vi "data_acquisition.vi"() -> ()   [LabVIEW 2020]
uses:
  <vilib>/regexp/Match Regular Expression.xnode
panel:
  in  "VISA resource name":refnum<visa-resource-name>="USB0::0x0471::0x2515::482A16001::INSTR"
  out "Resistance":dbl(graph)
  in  "measurement delay time (default 0.003)":dbl=0.003
  in  "Measurement speed":enum16{"FAST", "SLOW"}(ring)
  out "Samples / Second":dbl
  in  "measurement time":enum16{"FAST", "MED", "SLOW1", "SLOW2"}(ring)
  in  "Resistance measurement range":T1(ring)
  in  "Measurement mode":T2(ring)=enum."Resistance and Temp"
  in  "Display State":enum16{"Display ON", "Display OFF"}(ring)=enum."Display OFF"
  out "Temp":dbl
  out "Resistance":dbl format="%#_6p"
  out "read buffer":string
  in  "stop 2":bool
  out "error out":errorcluster
  # "Only 2 Ohm, 20 Ohm, 200 Ohm, 2 k \nare valid for  Measurement Mode at\nLow Voltage (LPR, LPR-T)"
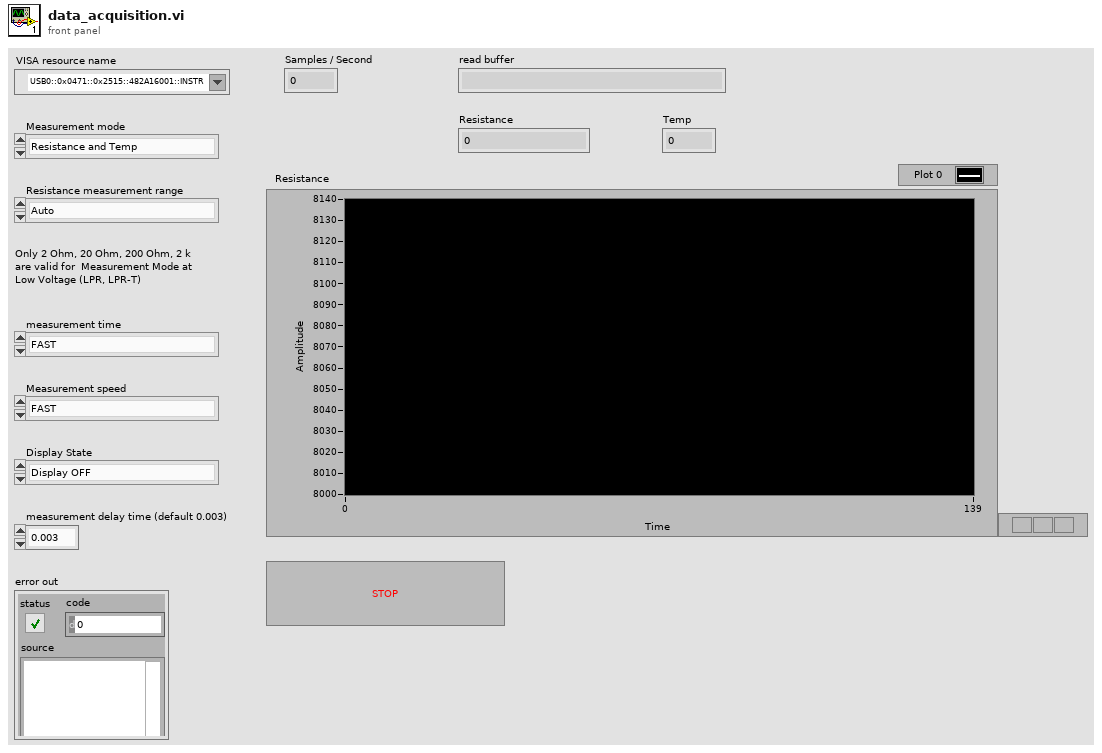
[diagram p1: front panel]
types:
  T1 = enum16{"Auto", "20 milli-Ohms", "200 milli-Ohms", "2 Ohms", "20 Ohms", "200 Ohms", "2 k-Ohms", "20 k-Ohms", "100 k-Ohms", "1 M-Ohms", "10 M-Ohms", "100 M-Ohms"}
  T2 = enum16{"Resistance", "Resistance and Temp", "Low Power Resistance", "Low Power Resisance and Temp", "Temp"}
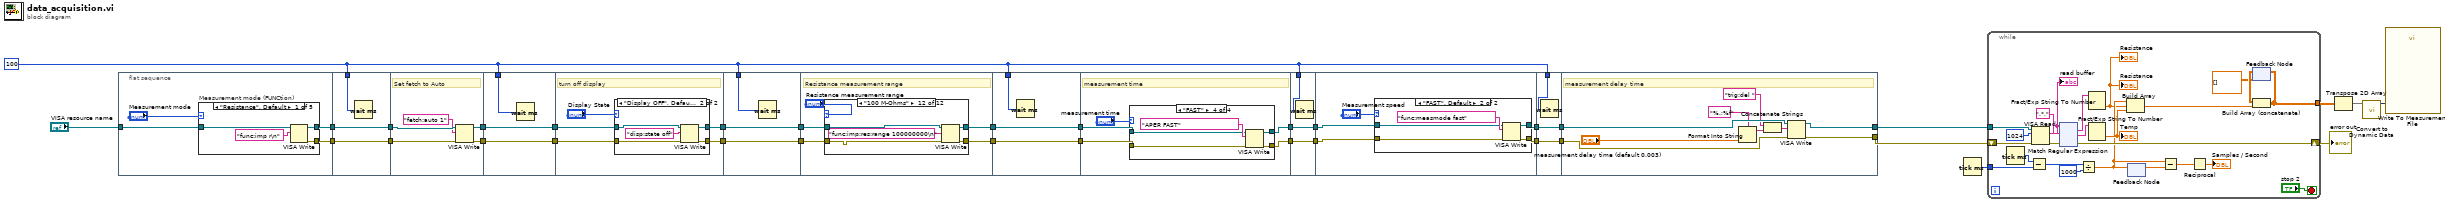
[diagram p0: block diagram]
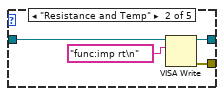
[diagram p2: hidden frame]
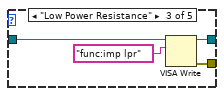
[diagram p3: hidden frame]
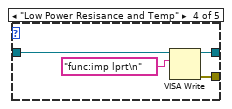
[diagram p4: hidden frame]
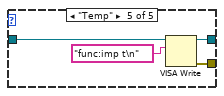
[diagram p5: hidden frame]
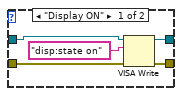
[diagram p6: hidden frame]
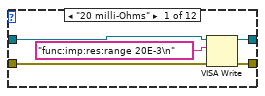
[diagram p7: hidden frame]
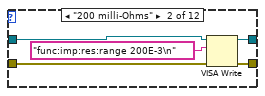
[diagram p8: hidden frame]
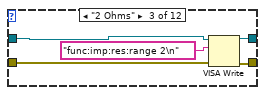
[diagram p9: hidden frame]
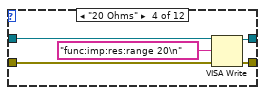
[diagram p10: hidden frame]
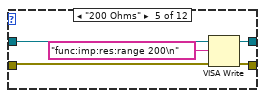
[diagram p11: hidden frame]
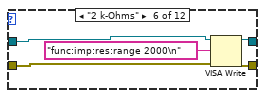
[diagram p12: hidden frame]
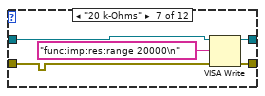
[diagram p13: hidden frame]
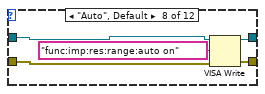
[diagram p14: hidden frame]
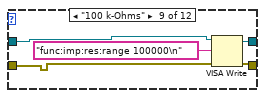
[diagram p15: hidden frame]
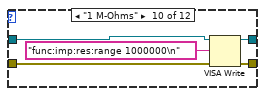
[diagram p16: hidden frame]
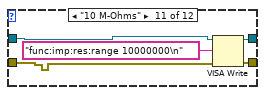
[diagram p17: hidden frame]
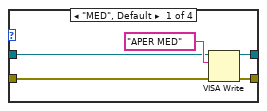
[diagram p18: hidden frame]
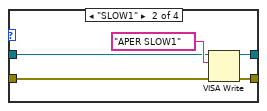
[diagram p19: hidden frame]
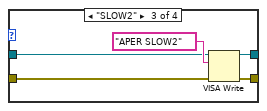
[diagram p20: hidden frame]
diagram:
  w1 = u32 100 ("delay before read (ms)")
  n1 = flat-sequence {
    tunnel: "VISA resource name" -> [w36]
    tunnel: [w34] -> w18
    tunnel: [w35] -> w17
    tunnel: [w60] -> w26
    tunnel: [w59] -> w25
    tunnel: w18 -> [w60]
    tunnel: w17 -> [w59]
    tunnel: w1 -> [w58]
    tunnel: w26 -> [w65]
    tunnel: w25 -> [w64]
    tunnel: [w63] -> w24
    tunnel: [w62] -> w23
    tunnel: w24 -> [w68]
    tunnel: w23 -> [w67]
    tunnel: w1 -> [w66]
    tunnel: [w68] -> w22
    tunnel: [w67] -> w21
    tunnel: w22 -> [w70]
    tunnel: w21 -> [w73]
    tunnel: [w72] -> w20
    tunnel: [w71] -> w19
    tunnel: w20 -> [w85]
    tunnel: w1 -> [w84]
    tunnel: w19 -> [w86]
    tunnel: [w86] -> w15
    tunnel: [w85] -> w14
    tunnel: w15 -> [w89]
    tunnel: w14 -> [w90]
    tunnel: [w87] -> w13
    tunnel: [w88] -> w12
    tunnel: w13 -> [w154]
    tunnel: w12 -> [w153]
    tunnel: [w154] -> w11
    tunnel: [w153] -> w10
    tunnel: w1 -> [w152]
    tunnel: w11 -> [w157]
    tunnel: w10 -> [w158]
    tunnel: [w155] -> w9
    tunnel: [w156] -> w8
    tunnel: w9 -> [w182]
    tunnel: w8 -> [w181]
    tunnel: [w182] -> w7
    tunnel: [w181] -> w6
    tunnel: w1 -> [w180]
    tunnel: w7 -> [w185]
    tunnel: w6 -> [w186]
    tunnel: [w184] -> w5
    tunnel: [w183] -> w4
    tunnel: w5 -> [w200]
    tunnel: w4 -> [w199]
    tunnel: [w200] -> w3
    tunnel: [w199] -> w2
    tunnel: w1 -> [w198]
    tunnel: [w206] -> w33
    tunnel: [w207] -> w32
    tunnel: w3 -> [w208]
    tunnel: w2 -> [w209]
    frame #0 {
      n2 = case "Measurement mode (FUNCtion)" shown="\"Resistance\", Default" "Measurement mode" {
        tunnel: w36 -> [w40 w45 w48 w52 w56]
        tunnel: [w39 w43 w47 w51 w55] -> w35
        tunnel: [w38 w42 w46 w50 w54] -> w34
        frame "Resistance", Default {
          n3 = VISA Write(VISA resource name=w40, write buffer="func:imp r\n") -> (VISA resource name out=w39:refnum<visa-resource-name>, error out=w38:errorcluster)  [unwired: 1 in, 1 out]
        }
        frame "Resistance and Temp" {
          n4 = VISA Write(VISA resource name=w45, write buffer="func:imp rt\n") -> (VISA resource name out=w43:refnum<visa-resource-name>, error out=w42:errorcluster)  [unwired: 1 in, 1 out]
        }
        frame "Low Power Resistance" {
          n5 = VISA Write(VISA resource name=w48, write buffer="func:imp lpr") -> (VISA resource name out=w47:refnum<visa-resource-name>, error out=w46:errorcluster)  [unwired: 1 in, 1 out]
        }
        frame "Low Power Resisance and Temp" {
          n6 = VISA Write(VISA resource name=w52, write buffer="func:imp lprt\n") -> (VISA resource name out=w51:refnum<visa-resource-name>, error out=w50:errorcluster)  [unwired: 1 in, 1 out]
        }
        frame "Temp" {
          n7 = VISA Write(VISA resource name=w56, write buffer="func:imp t\n") -> (VISA resource name out=w55:refnum<visa-resource-name>, error out=w54:errorcluster)  [unwired: 1 in, 1 out]
        }
      }
    }
    frame #1 {
      n8 = Wait (ms)(milliseconds to wait=w58) -> ()  [unwired: 1 out]
    }
    frame #2 {
      # "Set fetch to Auto"
      n9 = VISA Write(VISA resource name=w64, write buffer="fetch:auto 1", error in (no error)=w65) -> (VISA resource name out=w62:refnum<visa-resource-name>, error out=w63:errorcluster)  [unwired: 1 out]
    }
    frame #3 {
      n10 = Wait (ms)(milliseconds to wait=w66) -> ()  [unwired: 1 out]
    }
    frame #4 {
      # "turn off display"
      n11 = case shown="\"Display OFF\", Default" "Display State" {
        tunnel: w73 -> [w74 w82]
        tunnel: [w75 w81] -> w72
        tunnel: [w76 w80] -> w71
        tunnel: w70 -> [w77 w79]
        frame "Display ON" {
          n12 = VISA Write(VISA resource name=w74, write buffer="disp:state on", error in (no error)=w77) -> (VISA resource name out=w75:refnum<visa-resource-name>, error out=w76:errorcluster)  [unwired: 1 out]
        }
        frame "Display OFF", Default {
          n13 = VISA Write(VISA resource name=w82, write buffer="disp:state off", error in (no error)=w79) -> (VISA resource name out=w81:refnum<visa-resource-name>, error out=w80:errorcluster)  [unwired: 1 out]
        }
      }
    }
    frame #5 {
      n14 = Wait (ms)(milliseconds to wait=w84) -> ()  [unwired: 1 out]
    }
    frame #6 {
      # "Resistance measurement range"
      n15 = case shown="\"100 M-Ohms\"" "Resistance measurement range" {
        tunnel: w90 -> [w92 w100 w105 w108 w115 w117 w122 w127 w134 w137 w142 w148]
        tunnel: [w93 w99 w102 w110 w113 w120 w125 w130 w132 w140 w145 w150] -> w88
        tunnel: [w94 w98 w103 w109 w112 w119 w124 w129 w135 w139 w144 w149] -> w87
        tunnel: w89 -> [w95 w97 w104 w107 w114 w118 w123 w128 w133 w138 w143 w147]
        frame "20 milli-Ohms" {
          n16 = VISA Write(VISA resource name=w92, write buffer="func:imp:res:range 20E-3\n", error in (no error)=w95) -> (VISA resource name out=w93:refnum<visa-resource-name>, error out=w94:errorcluster)  [unwired: 1 out]
        }
        frame "200 milli-Ohms" {
          n17 = VISA Write(VISA resource name=w100, write buffer="func:imp:res:range 200E-3\n", error in (no error)=w97) -> (VISA resource name out=w99:refnum<visa-resource-name>, error out=w98:errorcluster)  [unwired: 1 out]
        }
        frame "2 Ohms" {
          n18 = VISA Write(VISA resource name=w105, write buffer="func:imp:res:range 2\n", error in (no error)=w104) -> (VISA resource name out=w102:refnum<visa-resource-name>, error out=w103:errorcluster)  [unwired: 1 out]
        }
        frame "20 Ohms" {
          n19 = VISA Write(VISA resource name=w108, write buffer="func:imp:res:range 20\n", error in (no error)=w107) -> (VISA resource name out=w110:refnum<visa-resource-name>, error out=w109:errorcluster)  [unwired: 1 out]
        }
        frame "200 Ohms" {
          n20 = VISA Write(VISA resource name=w115, write buffer="func:imp:res:range 200\n", error in (no error)=w114) -> (VISA resource name out=w113:refnum<visa-resource-name>, error out=w112:errorcluster)  [unwired: 1 out]
        }
        frame "2 k-Ohms" {
          n21 = VISA Write(VISA resource name=w117, write buffer="func:imp:res:range 2000\n", error in (no error)=w118) -> (VISA resource name out=w120:refnum<visa-resource-name>, error out=w119:errorcluster)  [unwired: 1 out]
        }
        frame "20 k-Ohms" {
          n22 = VISA Write(VISA resource name=w122, write buffer="func:imp:res:range 20000\n", error in (no error)=w123) -> (VISA resource name out=w125:refnum<visa-resource-name>, error out=w124:errorcluster)  [unwired: 1 out]
        }
        frame "Auto", Default {
          n23 = VISA Write(VISA resource name=w127, write buffer="func:imp:res:range:auto on", error in (no error)=w128) -> (VISA resource name out=w130:refnum<visa-resource-name>, error out=w129:errorcluster)  [unwired: 1 out]
        }
        frame "100 k-Ohms" {
          n24 = VISA Write(VISA resource name=w134, write buffer="func:imp:res:range 100000\n", error in (no error)=w133) -> (VISA resource name out=w132:refnum<visa-resource-name>, error out=w135:errorcluster)  [unwired: 1 out]
        }
        frame "1 M-Ohms" {
          n25 = VISA Write(VISA resource name=w137, write buffer="func:imp:res:range 1000000\n", error in (no error)=w138) -> (VISA resource name out=w140:refnum<visa-resource-name>, error out=w139:errorcluster)  [unwired: 1 out]
        }
        frame "10 M-Ohms" {
          n26 = VISA Write(VISA resource name=w142, write buffer="func:imp:res:range 10000000\n", error in (no error)=w143) -> (VISA resource name out=w145:refnum<visa-resource-name>, error out=w144:errorcluster)  [unwired: 1 out]
        }
        frame "100 M-Ohms" {
          n27 = VISA Write(VISA resource name=w148, write buffer="func:imp:res:range 100000000\n", error in (no error)=w147) -> (VISA resource name out=w150:refnum<visa-resource-name>, error out=w149:errorcluster)  [unwired: 1 out]
        }
      }
    }
    frame #7 {
      n28 = Wait (ms)(milliseconds to wait=w152) -> ()  [unwired: 1 out]
    }
    frame #8 {
      # "measurement time"
      n29 = case shown="\"FAST\"" "measurement time" {
        tunnel: w158 -> [w160 w168 w173 w175]
        tunnel: [w161 w167 w170 w178] -> w156
        tunnel: [w162 w166 w171 w177] -> w155
        tunnel: w157 -> [w163 w165 w172 w176]
        frame "MED", Default {
          n30 = VISA Write(VISA resource name=w160, write buffer="APER MED", error in (no error)=w163) -> (VISA resource name out=w161:refnum<visa-resource-name>, error out=w162:errorcluster)  [unwired: 1 out]
        }
        frame "SLOW1" {
          n31 = VISA Write(VISA resource name=w168, write buffer="APER SLOW1", error in (no error)=w165) -> (VISA resource name out=w167:refnum<visa-resource-name>, error out=w166:errorcluster)  [unwired: 1 out]
        }
        frame "SLOW2" {
          n32 = VISA Write(VISA resource name=w173, write buffer="APER SLOW2", error in (no error)=w172) -> (VISA resource name out=w170:refnum<visa-resource-name>, error out=w171:errorcluster)  [unwired: 1 out]
        }
        frame "FAST" {
          n33 = VISA Write(VISA resource name=w175, write buffer="APER FAST", error in (no error)=w176) -> (VISA resource name out=w178:refnum<visa-resource-name>, error out=w177:errorcluster)  [unwired: 1 out]
        }
      }
    }
    frame #9 {
      n34 = Wait (ms)(milliseconds to wait=w180) -> ()  [unwired: 1 out]
    }
    frame #10 {
      n35 = case shown="\"FAST\", Default" "Measurement speed" {
        tunnel: w186 -> [w191 w193]
        tunnel: [w190 w196] -> w183
        tunnel: [w189 w195] -> w184
        tunnel: w185 -> [w188 w194]
        frame "SLOW" {
          n36 = VISA Write(VISA resource name=w191, write buffer="func:measmode slow", error in (no error)=w188) -> (VISA resource name out=w190:refnum<visa-resource-name>, error out=w189:errorcluster)  [unwired: 1 out]
        }
        frame "FAST", Default {
          n37 = VISA Write(VISA resource name=w193, write buffer="func:measmode fast", error in (no error)=w194) -> (VISA resource name out=w196:refnum<visa-resource-name>, error out=w195:errorcluster)  [unwired: 1 out]
        }
      }
    }
    frame #11 {
      n38 = Wait (ms)(milliseconds to wait=w198) -> ()  [unwired: 1 out]
    }
    frame #12 {
      # "measurement delay time"
      n39 = Format Into String(format string="%.;%f", "measurement delay time (default 0.003)") -> (resulting string=w202:string)  [unwired: 2 in, 1 out]
      n40 = Concatenate Strings("trig:del " ("write buffer"), w202) -> (w201:string)
      n41 = VISA Write(VISA resource name=w209, write buffer=w201, error in (no error)=w208) -> (VISA resource name out=w206:refnum<visa-resource-name>, error out=w207:errorcluster)  [unwired: 1 out]
    }
  }
  n42 = Tick Count (ms)() -> (millisecond timer value=w30:u32)
  n43 = while {
    tunnel: w33 -> [w232]
    shift-right: [w225] -> w31
    shift-left: w32 -> [w231]
    tunnel: w30 -> [w223]
    tunnel: [w217] -> w28
    stop <- "stop 2" stop-if-true
    n44 = Tick Count (ms)() -> (millisecond timer value=w222:u32)
    n45 = Subtract(x=w222, y=w223) -> (x-y=w216:u32)
    n46 = VISA Read(VISA resource name=w232, byte count=u32 1024, error in (no error)=w231) -> (read buffer=w224:string, error out=w226:errorcluster)  [unwired: 2 out]
    "read buffer" <- w224
    n47 = xnode "Match Regular Expression"("input string"=w224, "regular expression"=".*,", "error in"=w226) -> ("whole match"=w228:string, "after match"=w227:string, "error out"=w225:errorcluster)  [unwired: 3 in, 2 out]
    n48 = Divide(x=w216, y=u32 1000) -> (x/y=w214:dbl)
    n49 = Fract/Exp String To Number(string=w228) -> (number=w210:dbl)  [unwired: 3 in, 1 out]
    "Resistance" <- w210
    "Resistance" <- w210
    n50 = Fract/Exp String To Number(string=w227) -> (number=w221:dbl)  [unwired: 3 in, 1 out]
    "Temp" <- w221
    n51 = Build Array(w214, w210, w221) -> (w220:dbl[])
    n52 = feedback #1() -> (w213:dbl)  [unwired: 1 in]
    n53 = feedback-in #1(w214) -> ()
    n54 = Subtract(x=w214, y=w213) -> (x-y=w212:dbl)
    n55 = Reciprocal(x=w212) -> (1/x=→"Samples / Second":dbl)
    n56 = feedback #2(dbl[][] []) -> (w219:dbl[][])
    n57 = Build Array (concatenate)(w219, w220) -> (w217:dbl[][])
    n58 = feedback-in #2(w217) -> ()
  }
  "error out" <- w31
  n59 = Transpose 2D Array(2D array=w28) -> (transposed array=w27:dbl[][])
  n60 = call "Convert to Dynamic Data"("2D Array"=w27) -> ("Dynamic Data Type"=w29:dynamicdata)  [unwired: 3 in]
  n61 = call "Write To Measurement File"("Signals"=w29) -> ()  [unwired: 16 in, 3 out]
